vi "Main.vi"() -> ()   [LabVIEW 2025]
uses:
  D:/LabVIEW Projects/Traffic-Light-Intersection-Project/Traffic Light--cluster.ctl
panel:
  in  "Stop Sequence":bool
  in  "Test All Lamps":bool
  in  "Launch Sequence":bool
  in  "Test West Green":bool
  in  "Test West Yellow":bool
  in  "Test West Red":bool
  in  "Test North Green":bool
  in  "Test North Yellow":bool
  in  "Test North Red":bool
  in  "Exit":bool
  out "West":T1
  out "North":T1
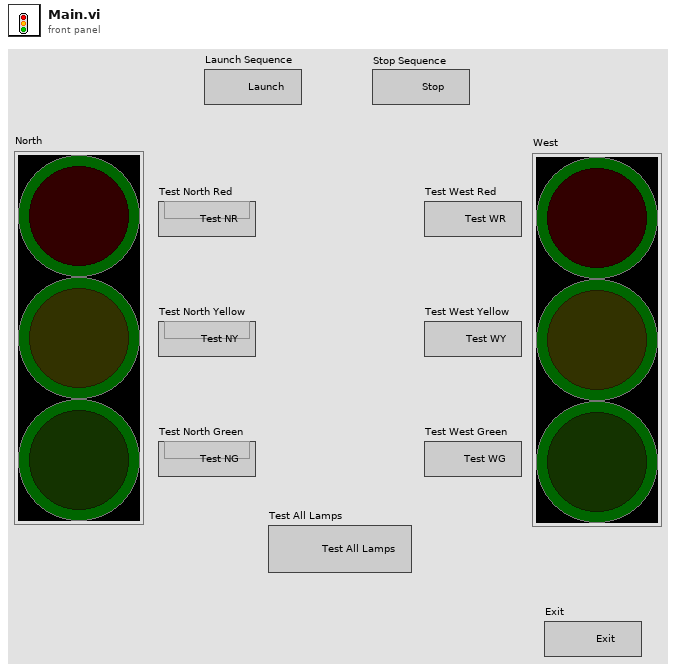
[diagram p1: front panel]
types:
  T1 = typedef "Traffic Light--cluster.ctl" = cluster{"Red":bool, "Yellow":bool, "Green":bool}
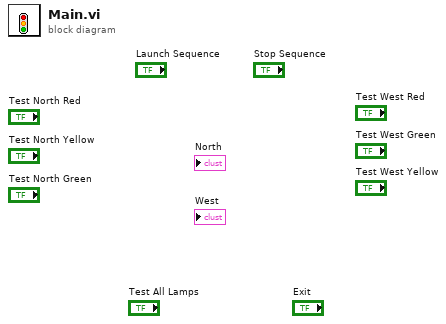
[diagram p0: block diagram]
diagram:
